vi "Cross-correlation function (for std. errs.)_PN.vi"(4 "Shift in":dbl[](array[numeric]), 5 "Current Block No":i32, 6 "V (m/s)":dbl[](array[numeric]), 7 "U (m/s)":dbl[](array[numeric])) -> (0 "Shift Out":dbl[](array[numeric]), 3 "Cross-correlation function":dbl[](array[numeric]))   [LabVIEW 2016]
uses:
  <vilib>/Analysis/2dsp.llb/1D Cross Correlation (DBL).vi
  <vilib>/Analysis/NI_AALPro.lvlib
  <vilib>/Analysis/NI_AALBase.lvlib
panel:
  # "PN 25/11/2016"
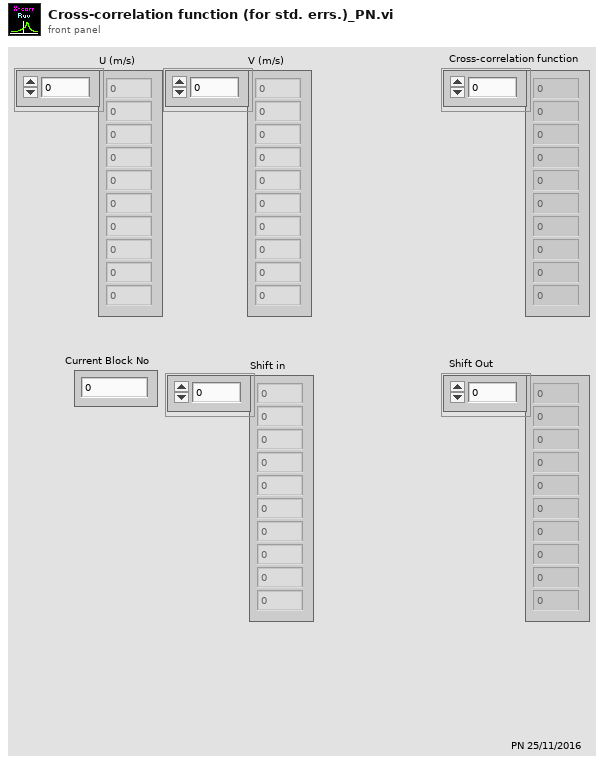
[diagram p1: front panel]
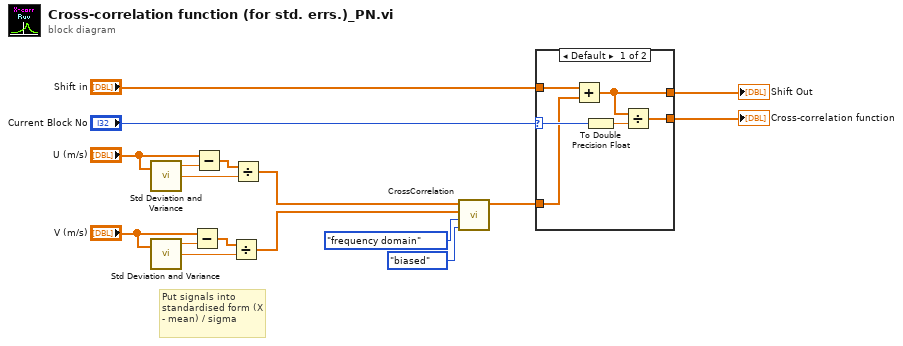
[diagram p0: block diagram]
diagram:
  # "Put signals into standardised form (X - mean) / sigma"
  n1 = call <vilib>:"Std Deviation and Variance.vi"("X"="U (m/s)") -> ("mean"=w12:dbl, "standard deviation"=w7:dbl)  [unwired: 1 in, 1 out]
  n2 = call <vilib>:"Std Deviation and Variance.vi"("X"="V (m/s)") -> ("mean"=w11:dbl, "standard deviation"=w8:dbl)  [unwired: 1 in, 1 out]
  n3 = Subtract(x="V (m/s)", y=w11) -> (x-y=w5:dbl[])
  n4 = Subtract(x="U (m/s)", y=w12) -> (x-y=w6:dbl[])
  n5 = Divide(x=w5, y=w8) -> (x/y=w3:dbl[])
  n6 = Divide(x=w6, y=w7) -> (x/y=w4:dbl[])
  n7 = call-poly <vilib>:"CrossCorrelation.vi"("normalization"=enum32{"none", "unbiased", "biased"}."biased", "algorithm"=enum32{"direct", "frequency domain"}."frequency domain", "Y"=w3, "X"=w4) -> ("Rxy"=w15:dbl[])  [unwired: 6 in, 1 out]
  n8 = case shown="Default" "Current Block No" {
    selector: "Current Block No" -> [w22 _]
    tunnel: [w23 w24] -> w13
    tunnel: w15 -> [w19 w24]
    tunnel: [w21 w24] -> w14
    tunnel: "Shift in" -> [w20 _]
    frame Default {
      n9 = Add(x=w20, y=w19) -> (x+y=w23:dbl[])
      n10 = To Double Precision Float(number=w22) -> (double precision float=w18:dbl)
      n11 = Divide(x=w23, y=w18) -> (x/y=w21:dbl[])
    }
    frame 1 {
    }
  }
  "Cross-correlation function" <- w14
  "Shift Out" <- w13
